vi "Add FPGA Hardware.vi"(7 "Overwrite Existing?":bool=TRUE, 8 "error in (no error)":errorcluster, 9 "FPGA Settings":T1={"Path"=path "", "RIO Name"="RIO0", "Aliases"=[]}, 10 "Base Node Path":string, 11 "SysDef Ref":T2) -> (0 "error out":errorcluster, 2 "New Node Path":string, 3 "SysDef Ref Out":T2)   [LabVIEW 2019, in "Simple SysDef API.lvlib"]
uses:
  <userlib>/SimpleSysDef/Simple SysDef API.lvlib
  <userlib>/SimpleSysDef/_SubVIs/System Definition Reference.ctl
  NationalInstruments.VeriStand.SystemDefinitionAPI
  <userlib>/SimpleSysDef/_SubVIs/Add FPGA Hardware_Settings.ctl
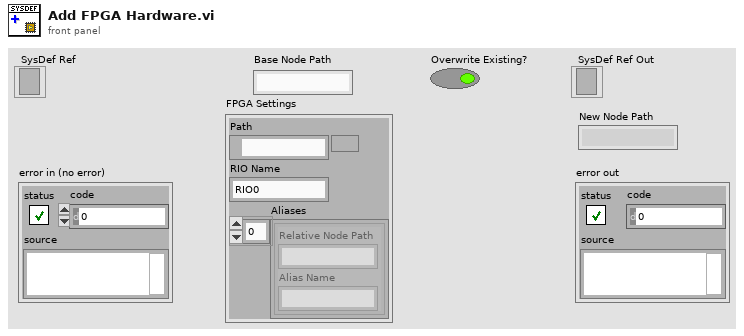
[diagram p1: front panel]
types:
  T1 = typedef "Simple SysDef API.lvlib/Add FPGA Hardware_Settings.ctl" = cluster{"Path":path, "RIO Name":string, "Aliases":cluster{"Relative Node Path":string, "Alias Name":string}[]}
  T2 = typedef "Simple SysDef API.lvlib/System Definition Reference.ctl" = refnum<k24>
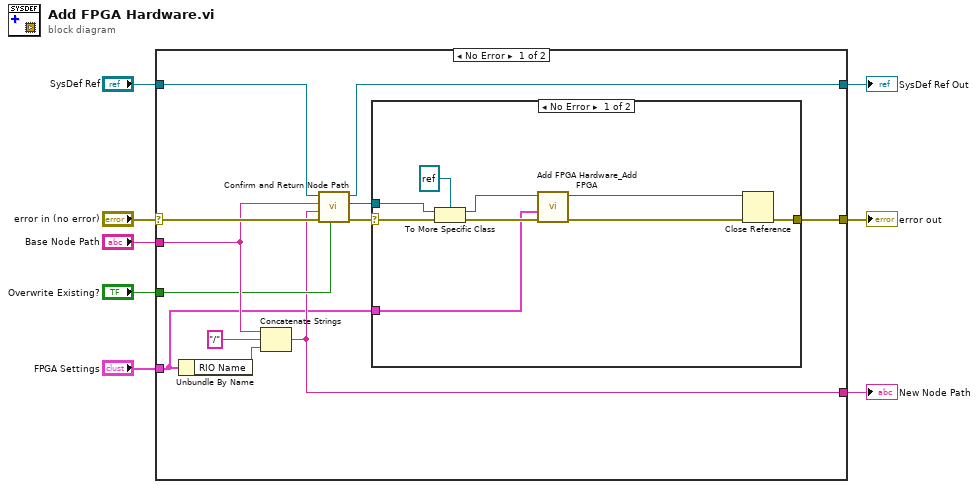
[diagram p0: block diagram]
diagram:
  n1 = case shown="No Error" "error in (no error)" {
    selector: "error in (no error)" -> [w20 w32]
    tunnel: [w15 w32] -> w7
    tunnel: "SysDef Ref" -> [w19 w31]
    tunnel: [w18 w31] -> w5
    tunnel: "Base Node Path" -> [w12 _]
    tunnel: "Overwrite Existing?" -> [w11 _]
    tunnel: "FPGA Settings" -> [w9 _]
    tunnel: [w10 _] -> w1
    frame No Error {
      n2 = Unbundle By Name(w9) -> ("RIO Name"=w16:string)
      n3 = Concatenate Strings(w12, "/" ("string"), w16) -> (w10:string)
      n4 = call <userlib>:"Confirm and Return Node Path.vi"("Overwrite Existing?"=w11, "error in (no error)"=w20, "New Node Path"=w10, "Base Node Path"=w12, "SysDef Ref"=w19) -> ("error out"=w13:errorcluster, "Node Ref"=w14:refnum<k24>, "SysDef Ref Out"=w18:T2)  [unwired: 4 in]
      n5 = case shown="No Error" w13 {
        selector: w13 -> [w28 w30]
        tunnel: [w27 w30] -> w15
        tunnel: w14 -> [w29 _]
        tunnel: w9 -> [w21 _]
        frame No Error {
          n6 = To More Specific Class(target class=refnum<k24> refnum ("Node Ref"), reference=w29, error in=w28) -> (specific class reference=w25:refnum<k24>, error out=w23:errorcluster)
          n7 = call <userlib>:"Add FPGA Hardware_Add FPGA.vi"("error in (no error)"=w23, "FPGA Settings"=w21, "FPGA Ref"=w25) -> ("error out"=w22:errorcluster, "FPGA Ref out"=w24:refnum<k24>)  [unwired: 7 in]
          n8 = Close Reference(reference=w24, error in (no error)=w22) -> (error out=w27:errorcluster)
        }
        frame Error {
        }
      }
    }
    frame Error {
    }
  }
  "SysDef Ref Out" <- w5
  "error out" <- w7
  "New Node Path" <- w1
